vi "Master Setup Check if References Changed.vi"(8 "Master Event Registration Refnum (in)":refnum<event-registration>, 11 "Pattern Label":T1 items=["Channel Setup (0)", "PID Setup (1)", "Filter Setup (2)", "~Reserved Old CAN Msgs (3)", "~Reserved Old CAN1 (4)", "~Reserved Old CAN2 (5)", "Digital Inputs Setup (6)", "Digital Outputs Setup (7)", "Logging 1 Setup (8)", "Logging 2 Setup (9)", "Logging 3 Setup (10)", "Setpoint Setup (11)", "Test Series Setup (12)", "Graph Setup (13)", "System Configure (14)", "Header (15)", "Profile Manager (16)", "Post-Mortem Logging (17)", "High-Speed Data (18)", "Statistic Channel Setup (19)", "Ramp Channel Setup (20)", "ETAS INCA Channel Setup (21)", "ETC ECCS Transducer Setup (22)", "ETC ECCS Test Setup (23)", "AVL AK Smoke Meter Setup (24)", "Triggers Setup (25)", "Alarm Limits Setup (26)", "YKWT1 Measurement (27)", "YKWT1 Instrument (28)", "Auto File Settings (29)", "Playback File Setting (30)", "UUT Constants (31)", "UPS Setup (32)", "Differential Channel Setup (33)", "Integral Channel Setup (34)", "Signal Channel Setup (35)", "Calibration Setup (36)", "BNC Setup (37)", "ASAP3 Setup (38)", "Chassis Force Calculations (39)", "Chassis Teststand Losses (40)", "Chassis Vehicle Losses (41)", "Formula Channels (42)", "ASAP3 Map Coords Setup (43)", "Digital Controls Setup (44)", "Push Buttons Setup (45)", "Sliders Setup (46)", "~Reserved~ (47)", "Email Setup (48)", "Timer Setup (49)", "Unit Conversion Setup (50)", "Visible Channels (51)", "Main Display Setup (52)", "Message Display Setup (53)", "Input Display Setup (54)", "Unico Parameter Downloads (55)", "Flow Meter Setup (56)", "Channel Zero Offset (57)", "YKWT2 Measurement (58)", "YKWT2 Instrument (59)", "~Reserved Old CAN3 (60)", "CAS Setup (61)", "Accumulation Channel Setup (62)", "Valvetrain Dynamics Setup (63)", "CCP Setup (64)", "System Log Setup (65)", "Throttle Controller (66)", "RE Shifter (67)", "Main Display (68)", "~Reserved~ (69)", "FlexRay (70)", "YKWT3 Measurement (71)", "YKWT3 Instrument (72)", "CAN XNET API (73)"]) -> (0 "Master Event Registration Refnum (out)":refnum<event-registration>)   [LabVIEW 2017]
uses:
  Master Setup Pattern Enum.ctl
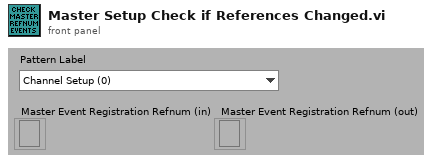
[diagram p1: front panel]
types:
  T1 = typedef "Master Setup Pattern Enum.ctl" = i32
  T2 = enum32{"invalid app kind", "Development System", "Run Time System", "Student Edition", "Embedded LabVIEW", "Evaluation", "Custom"}
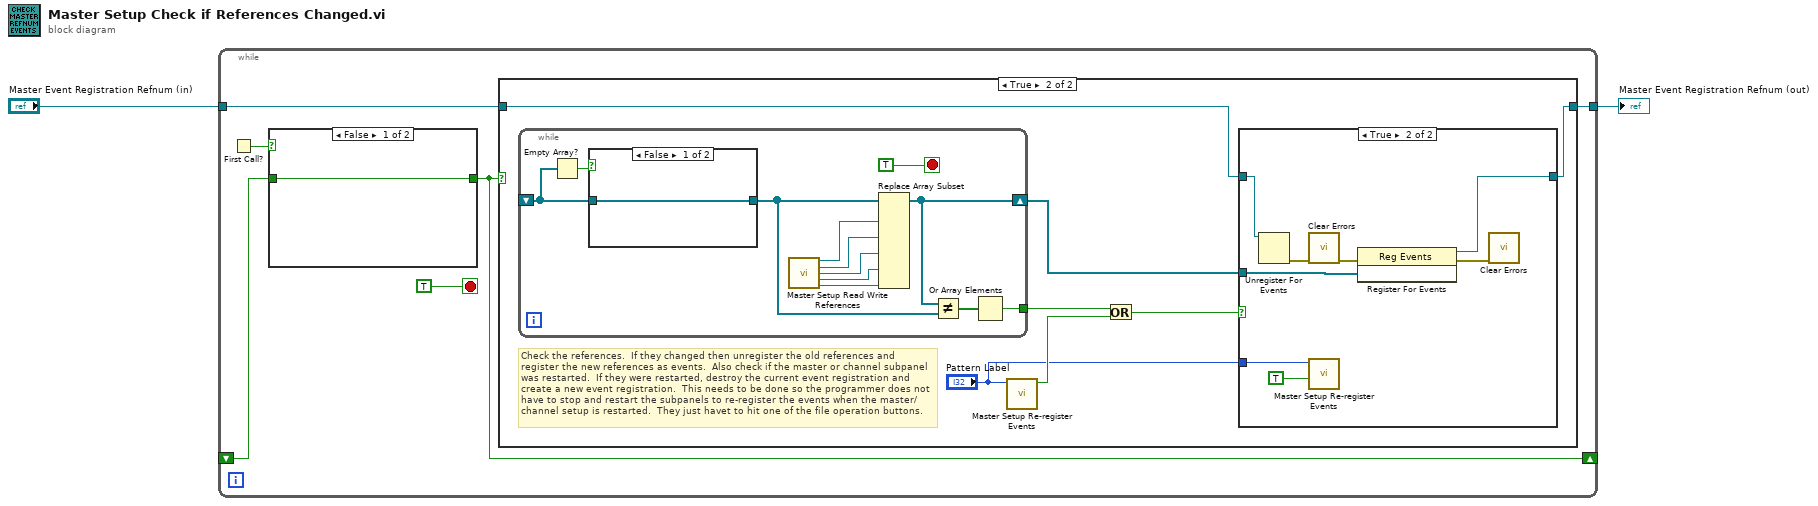
[diagram p0: block diagram]
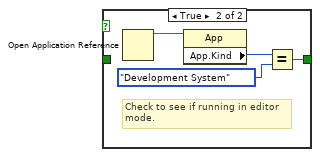
[diagram p2: hidden frame]
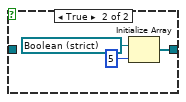
[diagram p5: hidden frame]
diagram:
  n1 = while {
    tunnel: [w8] -> w2
    tunnel: "Master Event Registration Refnum (in)" -> [w7]
    shift-right: [w5] -> _
    shift-left: _ -> [w4]
    stop <- TRUE stop-if-true
    n2 = First Call?() -> (First Call?: T/F=w6:bool)
    n3 = case shown="False" w6 {
      tunnel: [w9 w10] -> w5
      tunnel: w4 -> [w9 _]
      frame False {
      }
      frame True {
        # "Check to see if running in editor mode."
        n4 = Open Application Reference() -> (3:w13:refnum<vi>)  [unwired: 4 in, 1 out]
        n5 = property class="App"(reference=w13) -> ("App.Kind"=w11:T2)  [unwired: 1 in, 2 out]
        n6 = Equal?(x=w11, y=T2."Development System" ("Application:Kind")) -> (x = y?=w10:bool)
      }
    }
    n7 = case shown="True" w5 {
      tunnel: [w14 w19] -> w8
      tunnel: w7 -> [w14 w15]
      frame False {
      }
      frame True {
        # "Check the references.  If they changed then unregister the old references and register the new references as events.  Also check if the master or channel subpanel was restarted.  If they were restarted, destroy the current event registration and create a new event registration.  This needs to be done so the programmer does not have to stop and restart the subpanels to re-register the events when the master/channel setup is restarted.  They just havet to hit one of the file operation buttons."
        n8 = while {
          shift-right: [w41] -> w21
          shift-left: _ -> [w31]
          tunnel: [w38] -> w20
          stop <- TRUE stop-if-true
          n9 = Empty Array?(array=w31) -> (empty?=w32:bool)
          n10 = case shown="False" w32 {
            tunnel: [w43 w44] -> w39
            tunnel: w31 -> [w43 _]
            frame False {
            }
            frame True {
              n11 = Initialize Array(refnum<vi> refnum ("Update Channel Rings (out)"), 5 ("dimension size")) -> (w44:refnum<vi>[])
            }
          }
          n12 = call "Master Setup Read Write References.vi"() -> ("Master Exited (out)"=w33:refnum<vi>, "Master Open (out)"=w34:refnum<vi>, "Master Save (out)"=w35:refnum<vi>, "Update Channels (out)"=w36:refnum<vi>, "Update Channel Rings (out)"=w37:refnum<vi>)  [unwired: 10 in, 1 out]
          n13 = Replace Array Subset(array=w39, new element #1=w33, new element #2=w34, new element #3=w35, new element #4=w36, new element #5=w37) -> (w41:refnum<vi>[])  [unwired: 5 in]
          n14 = Not Equal?(x=w41, y=w39) -> (x != y?=w40:bool[])
          n15 = Or Array Elements(Boolean array=w40) -> (logical OR=w38:bool)
        }
        n16 = call "Master Setup Re-register Events.vi"("Pattern Label"="Pattern Label") -> ("Re-register Events"=w17:bool)  [unwired: 10 in]
        n17 = Or(x=w20, y=w17) -> (x .or. y?=w18:bool)
        n18 = case shown="True" w18 {
          tunnel: w21 -> [_ w30]
          tunnel: w15 -> [w22 w29]
          tunnel: [w22 w26] -> w19
          tunnel: "Pattern Label" -> [_ w24]
          frame False {
          }
          frame True {
            n19 = Unregister For Events(event registration refnum=w29) -> (error out=w28:errorcluster)  [unwired: 1 in]
            n20 = call <vilib>:"Clear Errors.vi"("error in (no error)"=w28) -> ("error out"=w27:errorcluster)  [unwired: 5 in, 1 out]
            n21 = call "Master Setup Re-register Events.vi"("Reset Register Events"=TRUE, "Pattern Label"=w24) -> ()  [unwired: 9 in, 1 out]
            n22 = register-events(error in=w27, w30) -> (reference out=w26:refnum<event-registration>, error out=w25:errorcluster)  [unwired: 1 in]
            n23 = call <vilib>:"Clear Errors.vi"("error in (no error)"=w25) -> ()  [unwired: 5 in, 2 out]
          }
        }
      }
    }
  }
  "Master Event Registration Refnum (out)" <- w2
